vi "Feeder Position.vi"(2 "Robot Mode":T1, 3 "setpoint":dbl format="%.2f", 4 "Z Axis":dbl) -> (0 "Rate":dbl, 1 "Finished":bool)   [LabVIEW 2012]
uses:
  <vilib>/Rock Robotics/WPI/DriverStation/WPI_DriverStationRobotMode.ctl
  typedefs/subStates.ctl
  <vilib>/addons/control/pid/pid.llb/PID (DBL).vi
  <vilib>/addons/control/pid/NI_PID_pid.lvlib
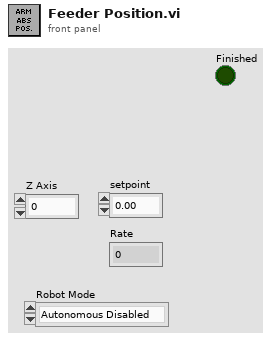
[diagram p1: front panel]
types:
  T1 = typedef "WPI_DriverStationRobotMode.ctl" = enum16{"Autonomous Disabled", "Autonomous Enabled", "Teleop Disabled", "Teleop Enabled", "Timeout", "Finish"}
  T2 = cluster{"proportional gain (Kc)":dbl, "integral time (Ti, min)":dbl, "derivative time (Td, min)":dbl}
  T3 = typedef "subStates.ctl" = enum16{"null", "wait", "driver control", "auto", "manual override", "hold position", "rotate", "feeder", "shoot", "end"}
  T4 = typedef "WPI_EncoderDevRef.ctl" = cluster{"DevStatus":errorcluster, "EncoderIndex":T5, "CounterIndex":T6, "DistancePerCount":dbl, "Decoding Type":T7}
  T5 = typedef "FPGA_EncoderIdx.ctl" = enum8{"Enc 0", "Enc 1", "Enc 2", "Enc 3", "Invalid"}
  T6 = typedef "FPGA_CounterCtrSystemIndex.ctl" = enum8{"Ctr 0", "Ctr 1", "Ctr 2", "Ctr 3", "Ctr 4", "Ctr 5", "Ctr 6", "Ctr 7", "Invalid"}
  T7 = typedef "WPI_EncoderType.ctl" = enum16{"1x", "2x", "4x"}
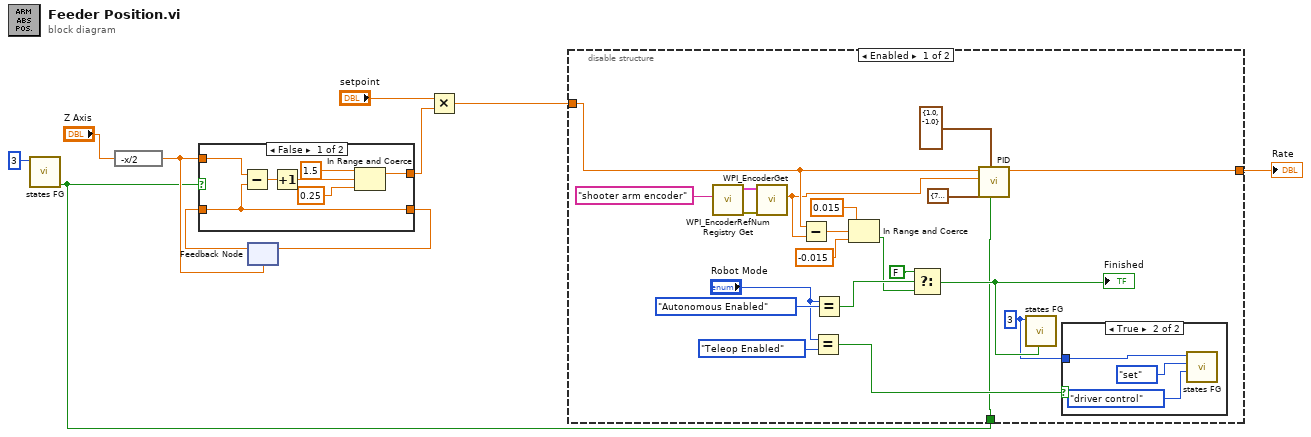
[diagram p0: block diagram]
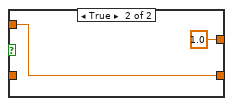
[diagram p2: hidden frame]
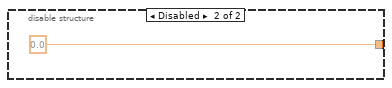
[diagram p4: hidden frame]
diagram:
  n1 = call "states FG.vi"("Loop ID"=3) -> ("first call?"=w1:bool)  [unwired: 7 in, 3 out]
  n2 = expression code="-x/2"("Z Axis") -> (w2:dbl)
  n3 = feedback #1(w2) -> (w6:dbl)
  n4 = case shown="False" w1 {
    tunnel: w2 -> [w17 w19]
    tunnel: [w16 w19] -> w7
    tunnel: w6 -> [w16 _]
    tunnel: [w13 1.0 ("upper limit")] -> w5
    frame False {
      n5 = Subtract(x=w17, y=w16) -> (x-y=w12:dbl)
      n6 = Increment(x=w12) -> (x+1=w11:dbl)
      n7 = In Range and Coerce(upper limit=1.5, x=w11, lower limit=0.25) -> (coerced(x)=w13:dbl)  [unwired: 1 out]
    }
    frame True {
    }
  }
  n8 = feedback-in #1(w7) -> ()
  n9 = Multiply(x="setpoint", y=w5) -> (x*y=w8:dbl)
  n10 = disable-structure shown="Enabled" {
    disable-tunnel: [w36 0.0 ("Rate")] -> w10
    disable-tunnel: w8 -> [w34 _]
    disable-tunnel: w1 -> [w20 _]
    frame Enabled {
      w22 = 3 ("Loop ID")
      n11 = call <vilib>:"WPI_EncoderRefNum Registry Get.vi"("refnum name"="shooter arm encoder") -> ("error out"=w40:errorcluster, "EncoderDevRef"=w39:T4)  [unwired: 9 in]
      n12 = call <vilib>:"WPI_EncoderGet.vi"("error in (no error)"=w40, "EncoderDevRef"=w39) -> ("Distance"=w26:dbl)  [unwired: 4 in, 5 out]
      n13 = Subtract(x=w34, y=w26) -> (x-y=w33:dbl)
      n14 = Equal?(x="Robot Mode", y=WPI_DriverStationRobotMode."Teleop Enabled") -> (x = y?=w21:bool)
      n15 = Equal?(x="Robot Mode", y=WPI_DriverStationRobotMode."Autonomous Enabled") -> (x = y?=w29:bool)
      n16 = In Range and Coerce(upper limit=0.015, x=w33, lower limit=-0.015) -> (In Range?=w28:bool)  [unwired: 1 out]
      n17 = Select(t=FALSE, s=w29, f=w28) -> (s? t:f=w25:bool)
      "Finished" <- w25
      n18 = call-poly <vilib>:"PID.vi"("reinitialize? (F)"=w20, "output range"=cluster{"output high":dbl, "output low":dbl} {"output high"=1.0, "output low"=-1.0}, "PID gains"=T2 {"proportional gain (Kc)"=7.0, "integral time (Ti, min)"=0.01, "derivative time (Td, min)"=0.0}, "process variable"=w26, "setpoint"=w34) -> ("output"=w36:dbl)  [unwired: 5 in, 1 out]
      n19 = call "states FG.vi"("exit in"=w25, "Loop ID"=w22) -> ()  [unwired: 6 in, 4 out]
      n20 = case shown="True" w21 {
        tunnel: w22 -> [_ w43]
        frame False {
        }
        frame True {
          n21 = call "states FG.vi"("subState in"=subStates."driver control", "menu (get)"=enum16{"set", "get"}."set", "Loop ID"=w43) -> ()  [unwired: 5 in, 4 out]
        }
      }
    }
    frame Disabled {
    }
  }
  "Rate" <- w10
